vi "Pack Step Value.vi"(8 "error in (no error)":errorcluster, 10 "Value":string, 11 "Set O2 Valve STEP in":refnum<class "O2 Valve STEP.lvclass">) -> (0 "error out":errorcluster, 3 "Set O2 Valve STEP out":refnum<class "O2 Valve STEP.lvclass">)   [LabVIEW 2014, in "O2 Valve STEP.lvlib" / "O2 Valve STEP.lvclass"]
uses:
  O2 Valve STEP.lvclass
  O2 Valve STEP.lvclass/O2 Valve STEP.ctl
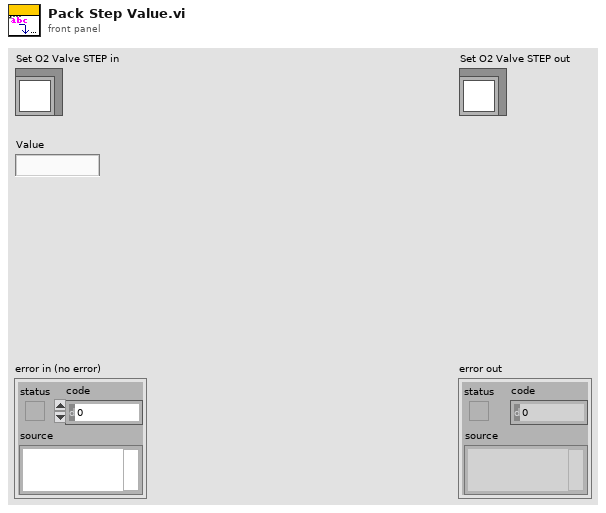
[diagram p1: front panel]
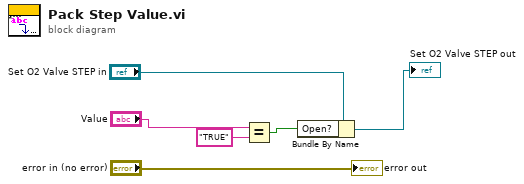
[diagram p0: block diagram]
diagram:
  n1 = Equal?(x="Value", y="TRUE") -> (x = y?=w2:bool)
  n2 = Bundle By Name(cluster="Set O2 Valve STEP in", "Open?"=w2) -> (→"Set O2 Valve STEP out":refnum<class "O2 Valve STEP.lvclass">)
  "error out" <- "error in (no error)"
